vi "Look_in_map_recursive.vi"(8 "Child Name":string, 9 "Child ID":string, 10 "Parent ID string":string, 11 "Map":map{string, cluster{string, variant}}(c390)) -> (2 "Parent in Maps":bool, 3 "Map Out":map{string, cluster{string, variant}}(c390))   [LabVIEW 2025]
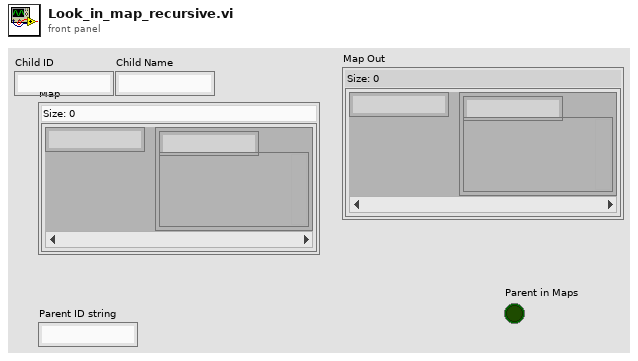
[diagram p1: front panel]
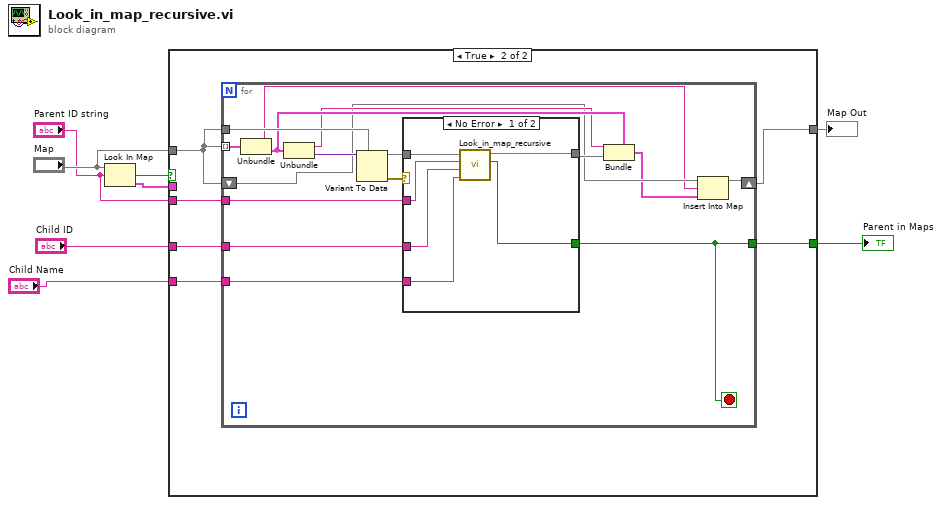
[diagram p0: block diagram]
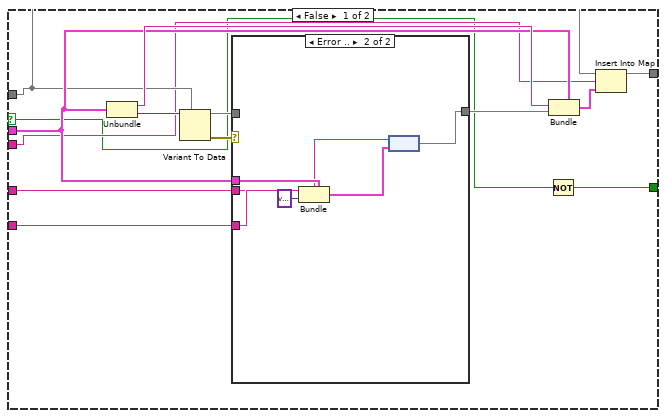
[diagram p2: hidden frame]
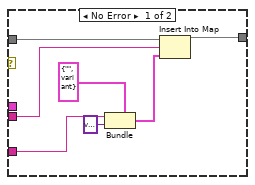
[diagram p3: hidden frame]
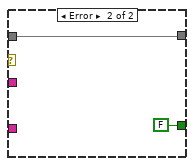
[diagram p4: hidden frame]
diagram:
  n1 = Look In Map(map="Map", key="Parent ID string") -> (key not found?=w8:bool, value=w4:cluster{string, variant})  [unwired: 1 in]
  n2 = case shown="True" w8 {
    selector: w8 -> [w10 _]
    tunnel: "Map" -> [w14 w38]
    tunnel: "Child ID" -> [w19 w41]
    tunnel: "Parent ID string" -> [w13 w40]
    tunnel: w4 -> [w16 _]
    tunnel: "Child Name" -> [w15 w39]
    tunnel: [w11 w37] -> w2
    tunnel: [w9 w36] -> w1
    frame False {
      n3 = Unbundle(w16) -> (w18:string, w22:variant)
      n4 = Variant To Data(type=w14, Variant=w22) -> (data=w20:map{string, cluster{string, variant}}, error out=w21:errorcluster)  [unwired: 1 in]
      n5 = case shown="Error .." w21 {
        tunnel: w20 -> [w29 _]
        tunnel: w19 -> [w28 w30]
        tunnel: [w24 w32] -> w17
        tunnel: w15 -> [w23 w34]
        tunnel: w16 -> [_ w33]
        frame No Error {
          n6 = Bundle(cluster=cluster{string, variant} {"", variant} ("value"), w23, variant) -> (w26:cluster{string, variant})
          n7 = Insert Into Map(map in=w29, key=w28, value=w26) -> (map out=w24:map{string, cluster{string, variant}})  [unwired: 2 out]
        }
        frame Error {
          n8 = Bundle(cluster=w33, w34, variant) -> (w31:cluster{string, variant})
          n9 = node(w30, w31) -> (w32:map{string, cluster{string, variant}})
        }
      }
      n10 = Not(x=w10) -> (.not. x?=w9:bool)
      n11 = Bundle(cluster=w16, w18, w17) -> (w12:cluster{string, variant})
      n12 = Insert Into Map(map in=w14, key=w13, value=w12) -> (map out=w11:map{string, cluster{string, variant}})  [unwired: 2 out]
    }
    frame True {
      n13 = for {
        tunnel: w38 -> [w47] mode=indexing
        tunnel: w38 -> [w57]
        tunnel: w41 -> [w53]
        tunnel: w40 -> [w52]
        tunnel: w39 -> [w51]
        shift-right: [w45] -> w37
        shift-left: w38 -> [w46]
        tunnel: [w42] -> w36
        stop <- w42 stop-if-true
        n14 = Unbundle(w47) -> (w44:string, w50:cluster{string, variant})
        n15 = Unbundle(w50) -> (w49:string, w55:variant)
        n16 = Variant To Data(type=w57, Variant=w55) -> (data=w54:map{string, cluster{string, variant}}, error out=w56:errorcluster)  [unwired: 1 in]
        n17 = case shown="No Error" w56 {
          tunnel: w54 -> [w63 w65]
          tunnel: w53 -> [w62 _]
          tunnel: w52 -> [w61 _]
          tunnel: w51 -> [w60 _]
          tunnel: [w59 w65] -> w48
          tunnel: [w58 FALSE ("Parent in Maps")] -> w42
          frame No Error {
            n18 = call "Look_in_map_recursive.vi"("Child Name"=w60, "Child ID"=w62, "Parent ID string"=w61, "Map"=w63) -> ("Parent in Maps"=w58:bool, "Map Out"=w59:map{string, cluster{string, variant}})  [unwired: 6 in]
          }
          frame Error {
          }
        }
        n19 = Bundle(cluster=w50, w49, w48) -> (w43:cluster{string, variant})
        n20 = Insert Into Map(map in=w46, key=w44, value=w43) -> (map out=w45:map{string, cluster{string, variant}})  [unwired: 2 out]
      }
    }
  }
  "Map Out" <- w2
  "Parent in Maps" <- w1
